vi "ImageReInitParams.vi"(0 "Image in":refnum<class "Image.lvclass">, 11 "error in (no error)":errorcluster) -> (4 "Image out":refnum<class "Image.lvclass">, 15 "error out":errorcluster)   [LabVIEW 2012, in "Image.lvclass"]
uses:
  classes/Image.lvclass
  classes/Image.lvclass/Image.ctl
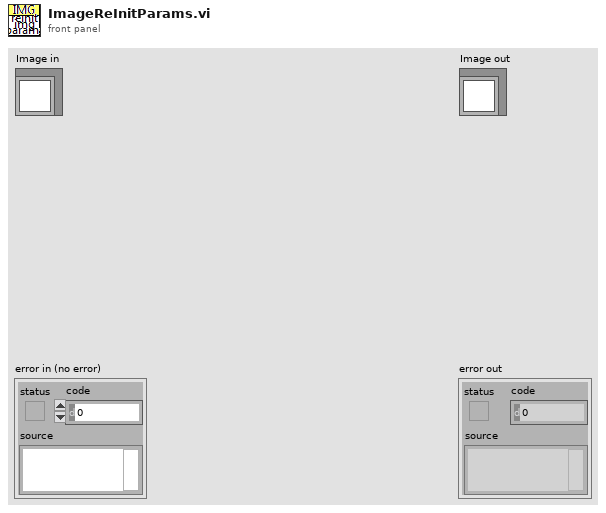
[diagram p1: front panel]
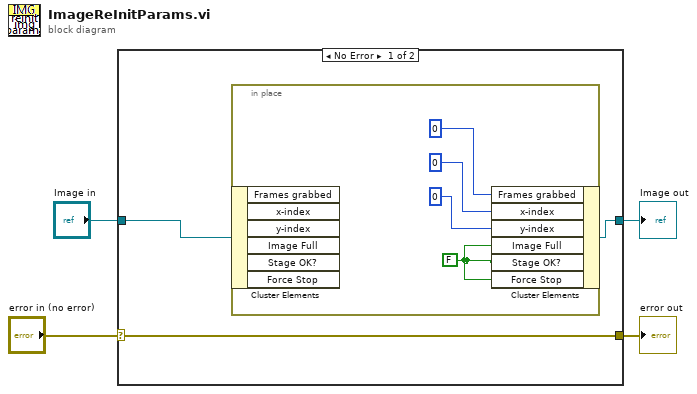
[diagram p0: block diagram]
diagram:
  n1 = case shown="No Error" "error in (no error)" {
    selector: "error in (no error)" -> [w7 w13]
    tunnel: [w7 w13] -> w3
    tunnel: [w5 w12] -> w1
    tunnel: "Image in" -> [w6 w12]
    frame No Error {
      n2 = in-place {
        w8 = FALSE
        n3 = in-place-cluster #1(w6) -> ()  [unwired: 6 out]
        n4 = in-place-cluster #1("Frames grabbed"=0, "x-index"=0, "y-index"=0, "Image Full"=w8, "Stage OK?"=w8, "Force Stop"=w8) -> (w5:refnum<class "Image.lvclass">)
      }
    }
    frame Error {
    }
  }
  "error out" <- w3
  "Image out" <- w1
